vi "Untitled 2.vi"() -> ()   [LabVIEW 2020]
uses:
  <vilib>/Utility/Data Type/Type Definitions/Data Type.ctl
  <vilib>/Utility/Data Type/Type Definitions/Type Definition Info.ctl
  Generate-Go-CMD/TestTD.ctl
  <vilib>/Utility/Data Type/NI_Data Type.lvlib
panel:
  out "Array 3":string[](array[string])
  out "Array 2":string[](array[string])
  out "Array":string[](array[string])
  in  "Cluster":T1
  out "type definition info":T2
  out "name":string
  out "type":T3
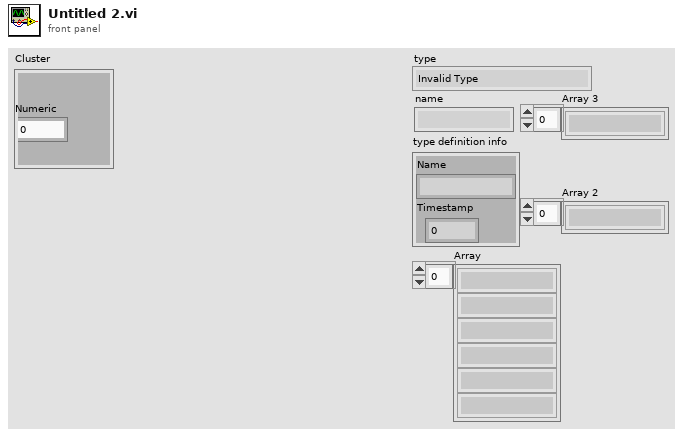
[diagram p1: front panel]
types:
  T1 = typedef "TestTD.ctl" = cluster{"Numeric":dbl}
  T2 = typedef "NI_Data Type.lvlib/Type Definition Info.ctl" = cluster{"Name":string, "Timestamp":u32}
  T3 = typedef "NI_Data Type.lvlib/Data Type.ctl" = enum8{"Invalid Type", "Void", "I8", "I16", "I32", "I64", "U8", "U16", "U32", "U64", "Single Float", "Double Float", "Extended Float", "Single Complex", "Double Complex", "Extended Complex", "Enum U8", "Enum U16", "Enum U32", "Enum U64", "Single Float With Unit", "Double Float With Unit", "Extended Float With Unit", "Single Complex with Unit", "Double Complex with Unit", "Extended Complex with Unit", "Boolean", "String", "Path", "Picture", "Tag", "Array", "Cluster", "Variant", "LV Variant", "Waveform", "Timestamp", "Digital Waveform", "Digital Data", "ExpressData", "Refnum", "External Data", "VI", "Poly VI", "LabVIEW Class Instance", "Fixed Point", "Set Collection", "Map Collection"}
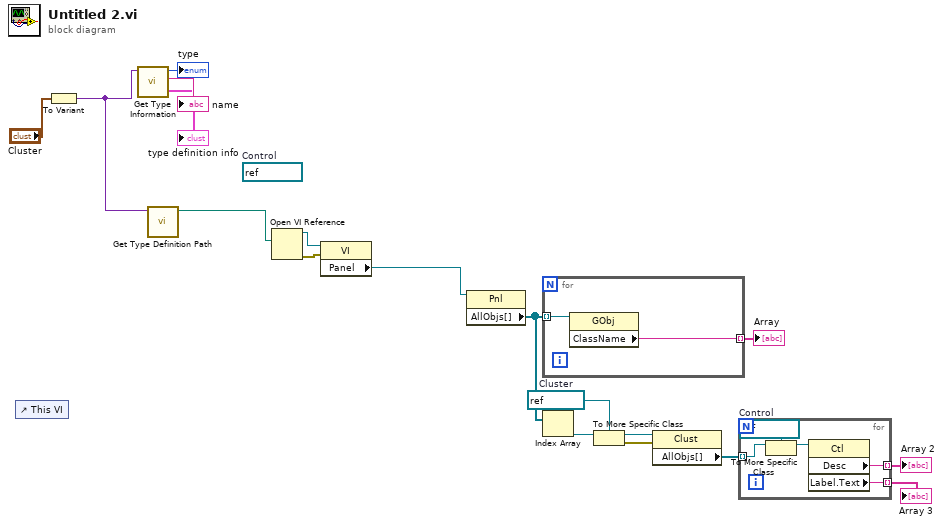
[diagram p0: block diagram]
diagram:
  w6 = refnum<vi> refnum  # Cluster
  (unwired) refnum<vi> refnum  # Control
  n1 = control-ref of="This VI"() -> ()  [unwired: 1 out]
  n2 = To Variant(anything="Cluster") -> (Variant=w14:variant)
  n3 = call <vilib>:"Get Type Information.vi"("variant"=w14) -> ("name"=→"name":string, "type"=→"type":T3, "type definition info"=→"type definition info":T2)  [unwired: 6 in, 2 out]
  n4 = call <vilib>:"Get Type Definition Path.vi"("variant"=w14) -> ("type definition path"=w13:path)  [unwired: 9 in, 1 out]
  n5 = Open VI Reference(vi path=w13) -> (vi reference=w11:refnum<vi>, error out=w12:errorcluster)  [unwired: 5 in]
  n6 = property class="VI"(reference=w11, error in=w12) -> ("Panel"=w10:refnum<vi>)  [unwired: 2 out]
  n7 = property class="Pnl"(reference=w10) -> ("AllObjs[]"=w8:refnum<vi>[])  [unwired: 1 in, 2 out]
  n8 = for {
    tunnel: w8 -> [w20] mode=indexing
    tunnel: [w19] -> w9 mode=indexing
    n9 = property class="GObj"(reference=w20) -> ("ClassName"=w19:string)  [unwired: 1 in, 2 out]
  }
  "Array" <- w9
  n10 = Index Array(array=w8) -> (element=w7:refnum<vi>)  [unwired: 1 in]
  n11 = To More Specific Class(target class=w6, reference=w7) -> (specific class reference=w5:refnum<vi>, error out=w4:errorcluster)  [unwired: 1 in]
  n12 = property class="Clust"(reference=w5, error in=w4) -> ("AllObjs[]"=w3:refnum<vi>[])  [unwired: 2 out]
  n13 = for {
    tunnel: w3 -> [w24] mode=indexing
    tunnel: [w25] -> w2 mode=indexing
    tunnel: [w21] -> w1 mode=indexing
    w23 = refnum<vi> refnum  # Control
    n14 = To More Specific Class(target class=w23, reference=w24) -> (specific class reference=w22:refnum<vi>)  [unwired: 1 in, 1 out]
    n15 = property class="Ctl"(reference=w22) -> ("Desc"=w25:string, "Label.Text"=w21:string)  [unwired: 1 in, 2 out]
  }
  "Array 2" <- w2
  "Array 3" <- w1
